vi "FTW-Email-AddressValidator.vi"(0 "Email Address":string, 11 "error in":errorcluster) -> (15 "error out":errorcluster)   [LabVIEW 2015]
uses:
  regex/FTW-Regex-Execute.vi
  error/FTW-ERR-ThrowError.vi
  error/FTW-ERR-CallChain.vi
  error/FTW-ERR-NoErrorConstant.vi
  string/FTW-STR-ReplaceWhitespace.vi
  string/FTW-STR-Array-Delimit.vi
  regex/FTW-Regex-Construct.vi
  lib/FTW-KernelFilepath.vi
  regex/FTW-Regex-Destroy.vi
panel:
  # "Inputs"
  # "Outputs"
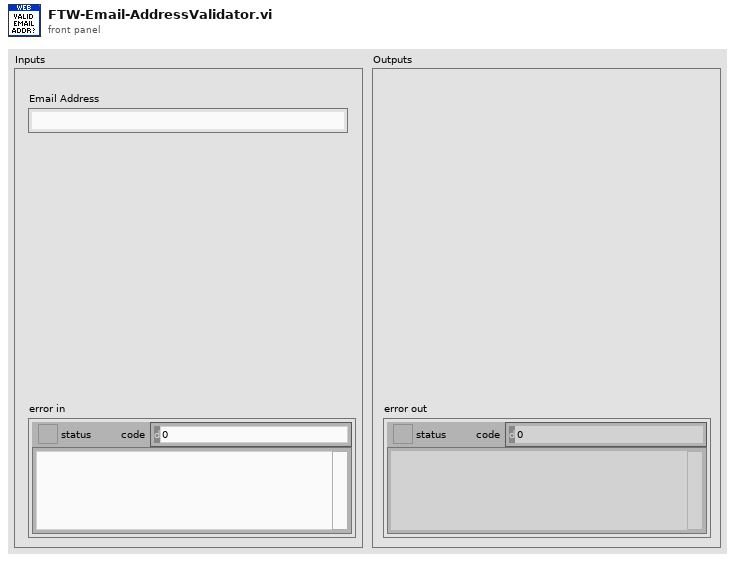
[diagram p1: front panel]
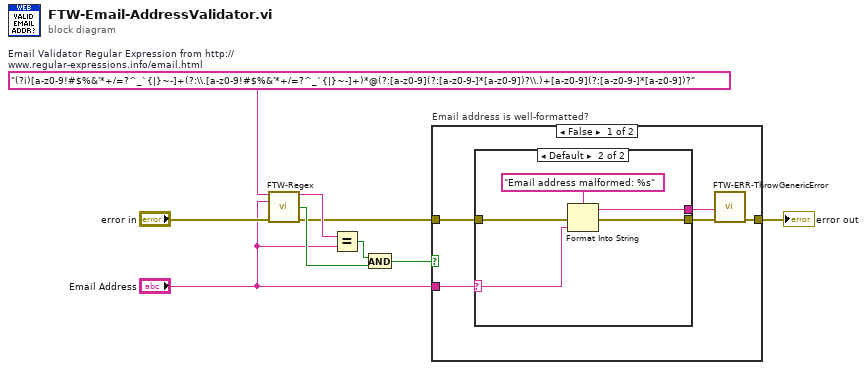
[diagram p0: block diagram]
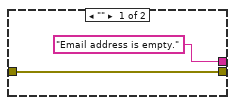
[diagram p2: hidden frame]
diagram:
  w9 = "(?i)[a-z0-9!#$%&'*+/=?^_`{|}~-]+(?:\\.[a-z0-9!#$%&'*+/=?^_`{|}~-]+)*@(?:[a-z0-9](?:[a-z0-9-]*[a-z0-9])?\\.)+[a-z0-9](?:[a-z0-9-]*[a-z0-9])?"  # Email Validator Regular Expression from http://www.regular-expressions.info/email.html
  n1 = call "FTW-Regex.vi"("Regular Expression"=w9, "Input String"="Email Address", "error in"="error in") -> ("Match"=w8:string, "Match Found?"=w6:bool, "error out"=w3:errorcluster)  [unwired: 8 in, 2 out]
  n2 = Equal?(x=w8, y="Email Address") -> (x = y?=w5:bool)
  n3 = And(x=w5, y=w6) -> (x .and. y?=w4:bool)
  n4 = case "Email address is well-formatted?" shown="False" w4 {
    tunnel: w3 -> [w12 w22]
    tunnel: [w11 w22] -> w2
    tunnel: "Email Address" -> [w10 _]
    frame False {
      n5 = case shown="Default" w10 {
        selector: w10 -> [_ w17]
        tunnel: [w16 w21] -> w14
        tunnel: ["Email address is empty." w20] -> w13
        tunnel: w12 -> [w16 w18]
        frame "" {
        }
        frame Default {
          n6 = Format Into String(format string="Email address malformed: %s" ("Error Message"), error in=w18, w17) -> (resulting string=w20:string, error out=w21:errorcluster)  [unwired: 1 in]
        }
      }
      n7 = call "FTW-ERR-ThrowGenericError.vi"("Error Message"=w13, "error in"=w14) -> ("error out"=w11:errorcluster)  [unwired: 13 in]
    }
    frame True {
    }
  }
  "error out" <- w2
